vi "File Load Dialog.vi"(6 "cycle range":u16=720, 8 "error in (no error)":errorcluster, 11 "Node Ptr":T4 format="%.0x") -> (0 "error out":errorcluster, 1 "Position reference":T1, 2 "Cancelled":bool, 3 "Data":dbl[](array[numeric]))   [LabVIEW 2013, in "Engine Simulation Toolkit System Explorer.lvlib"]
uses:
  Engine Simulation Toolkit System Explorer.lvlib
  FPGA Mem Size.ctl
  Position Reference.ctl
  Data Replay Data Selection Method.ctl
  <vilib>/NI Veristand/Custom Device API/Custom Device Item Ref.ctl
  Data File Loader/File Interface.lvlib
  <vilib>/NI Veristand/Custom Device API/Custom Device API.lvlib
panel:
  in  "DispTwoRotations":bool
  in  "ReverseData":bool
  in  "Missing teeth location (degrees)":dbl=1.0 min=0.0
  in  "Samples":i32=1 min=1
  in  "File start offset":i32=1 min=0
  in  "Data Selection Method":T2
  in  "DataPlugin":u16(ring)
  out "Loaded samples":i32=1 min=1
  out "Loaded start offset":i32=1 min=0
  in  "Channel":u16(ring)
  in  "Selected File":path
  in  "Group":u16(ring)
  in  "FPGA memory size":T3=enum."16,384"
  in  "CycleAngle?":T1 caption="Position reference"
  in  "Cancel":bool
  in  "OK":bool
  out "Data Graph":waveform(dbl)(graph)
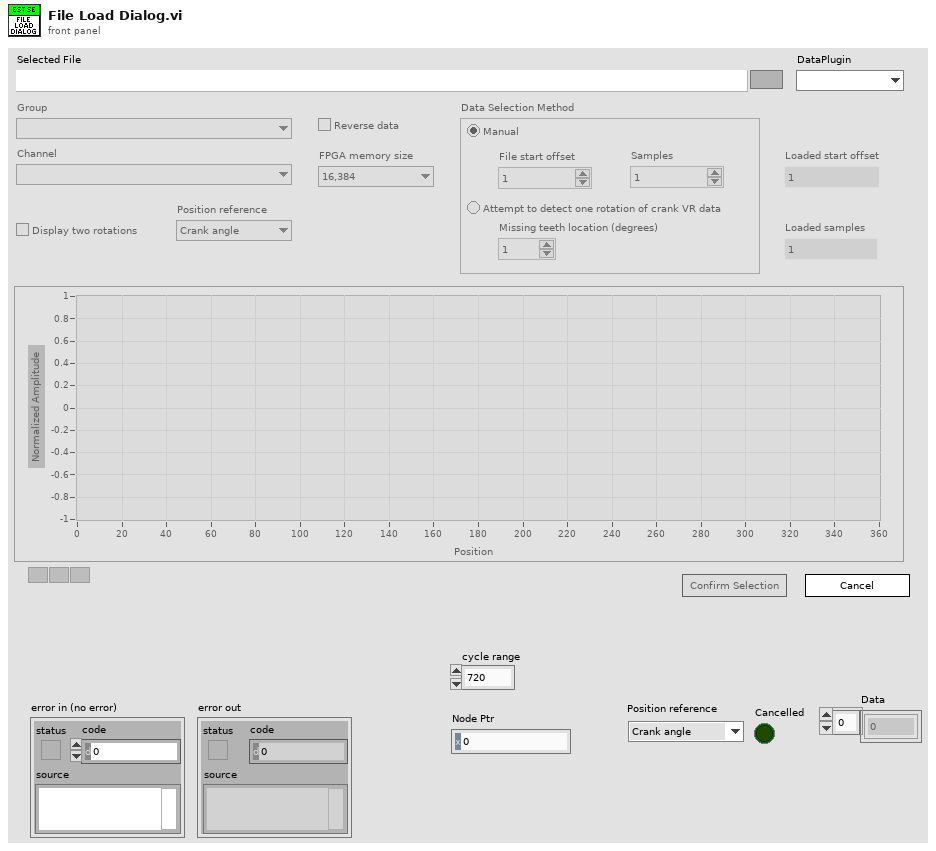
[diagram p1: front panel]
types:
  T1 = typedef "Engine Simulation Toolkit System Explorer.lvlib/Position Reference.ctl" = enum16{"Crank angle", "Cycle angle"}
  T2 = typedef "Engine Simulation Toolkit System Explorer.lvlib/Data Replay Data Selection Method.ctl" = enum32{"Manual", "AutoVRCrank"}
  T3 = typedef "Engine Simulation Toolkit System Explorer.lvlib/FPGA Mem Size.ctl" = enum16{"65,536", "32,768", "16,384", "8,192", "4,096", "2,048", "1,024"}
  T4 = typedef "Custom Device API.lvlib/Custom Device Item Ref.ctl" = u64
  T5 = typedef "Engine Simulation Toolkit System Explorer.lvlib/File Load Dialog.ctl" = cluster{"File":path, "Group":string, "Channel":string, "DataPlugin":string, "MissingTeeth":dbl, "ErrState":string, "File Selected":bool, "Data Selection Method":T2, "Offset":i32, "Length":i32, "DataPlugins Info":T6[], "Controls":refnum<vi>[], "File Ref":refnum<k20>, "Groups":string[], "Channels":string[], "Groups Refs":refnum<k20>[], "Channel Refs":refnum<k20>[], "Cancelled":bool, "Position reference":T1, "FPGA memory size":T3, "GroupRef":refnum<k20>, "ChanRef":refnum<k20>, "Data":dbl[], "ReverseData":bool, "DispTwoRotations":bool, "cycle range":u16}
  T6 = typedef "usiPluginInformation.ctl" = cluster{"name":string, "version":string, "type":string, "read-only?":bool, "extensions":string[]}
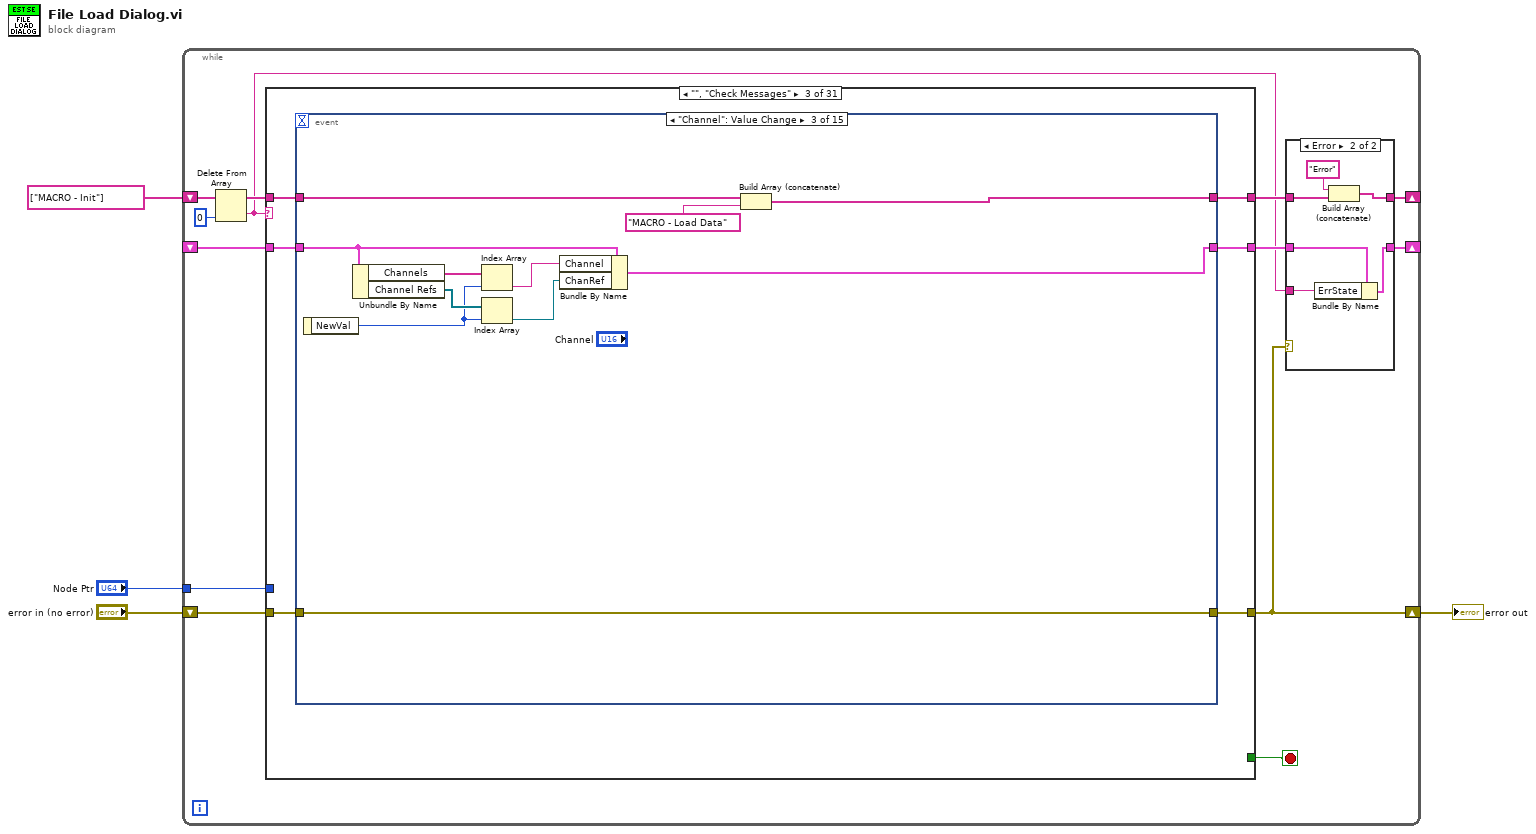
[diagram p0: block diagram]
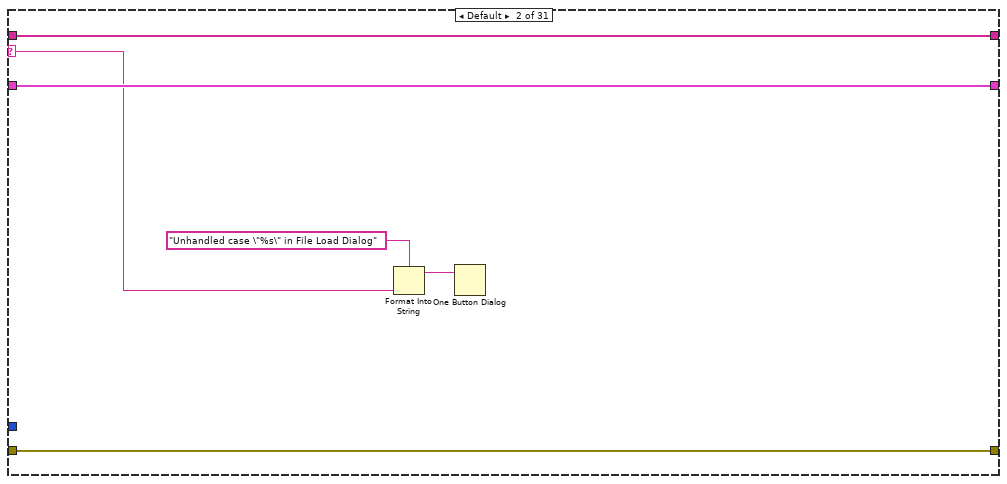
[diagram p4: hidden frame]
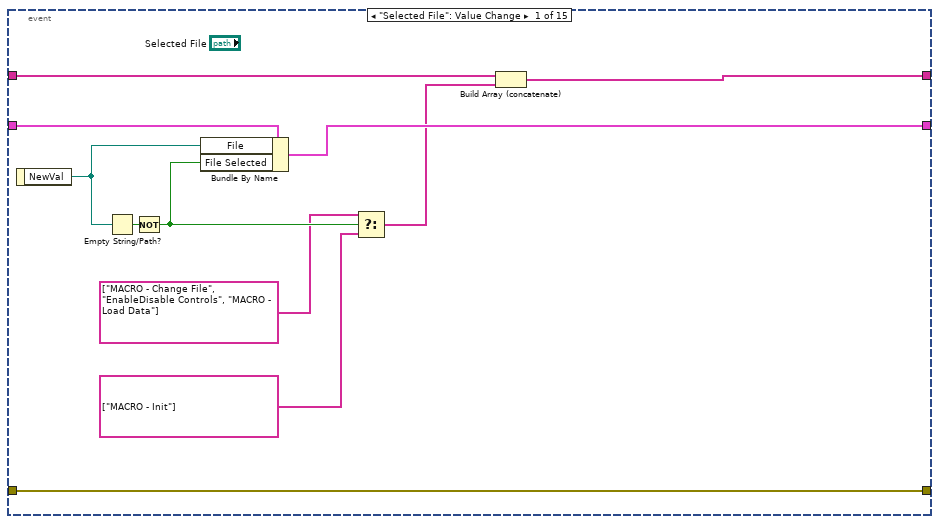
[diagram p5: hidden frame]
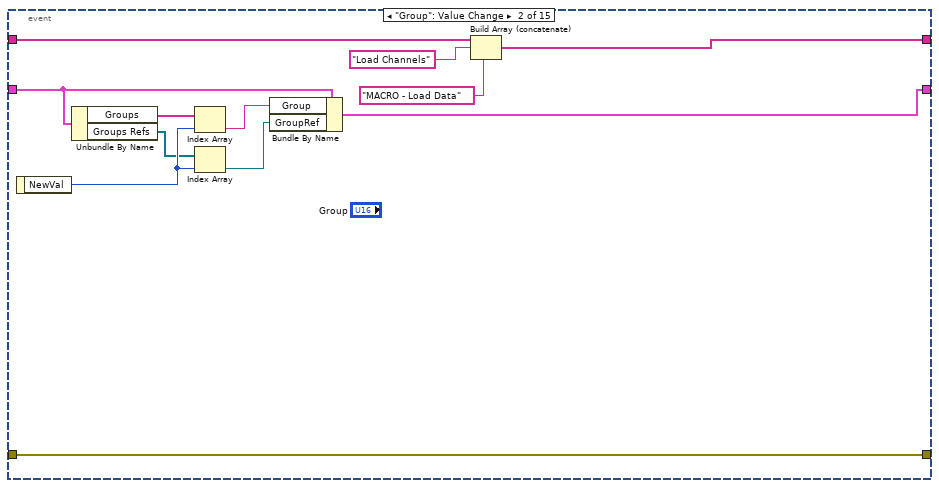
[diagram p6: hidden frame]
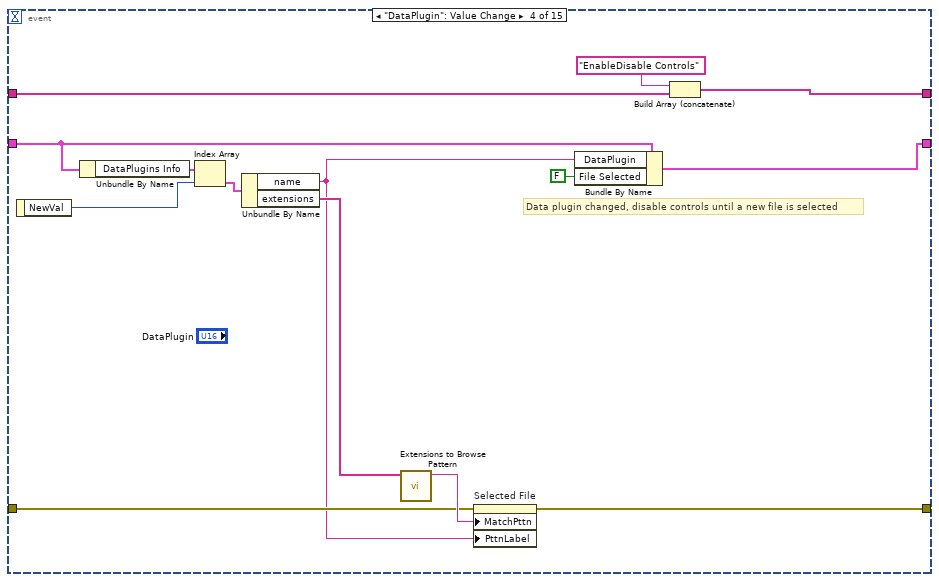
[diagram p7: hidden frame]
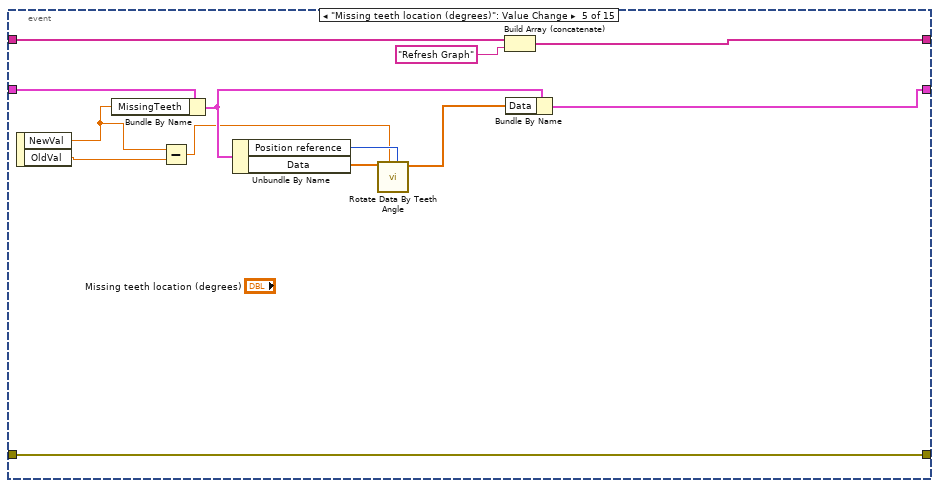
[diagram p8: hidden frame]
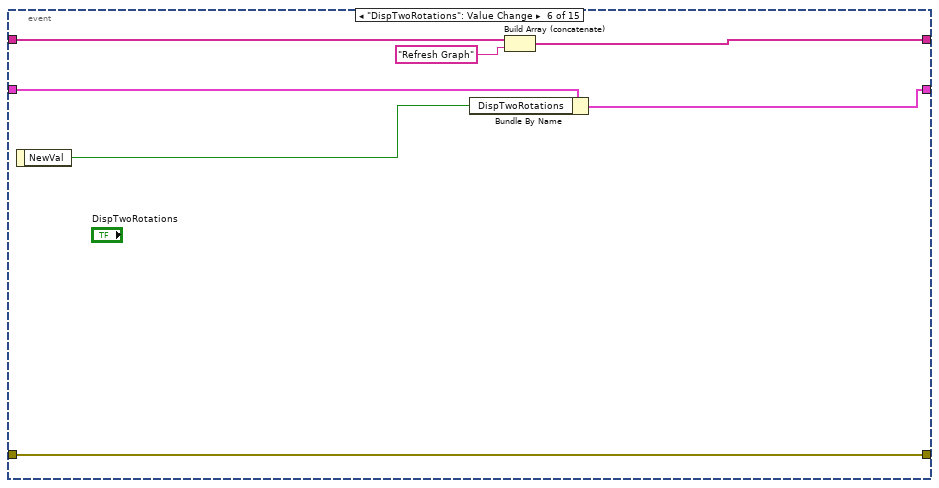
[diagram p9: hidden frame]
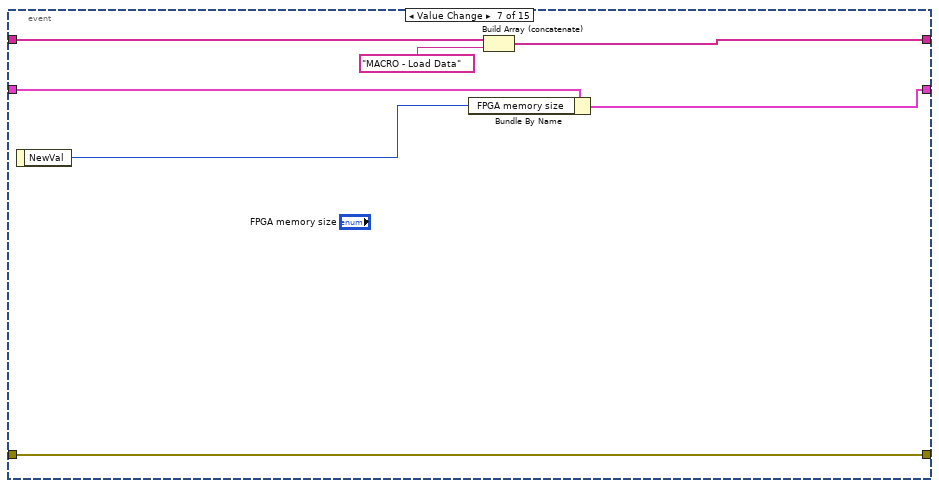
[diagram p10: hidden frame]
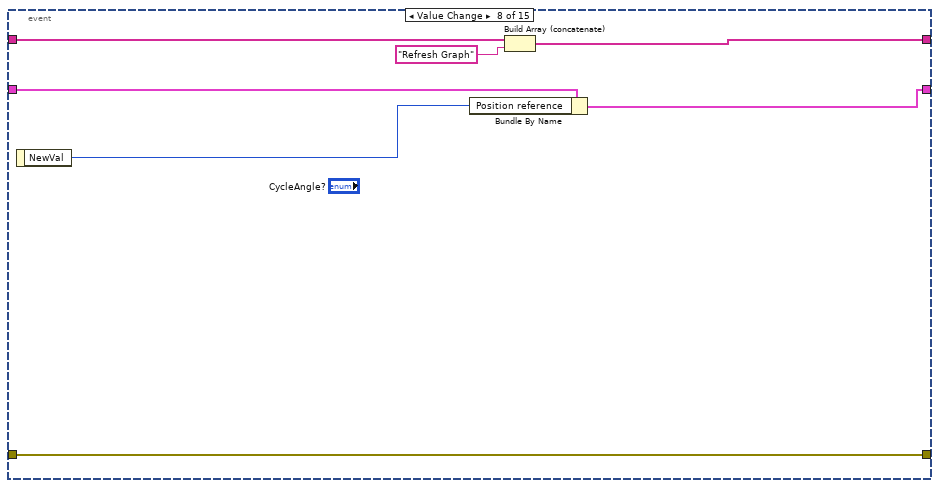
[diagram p11: hidden frame]
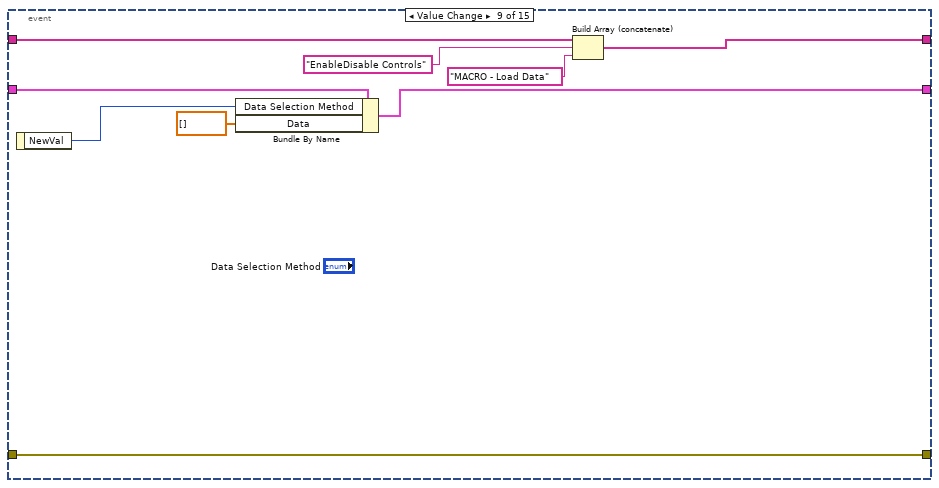
[diagram p12: hidden frame]
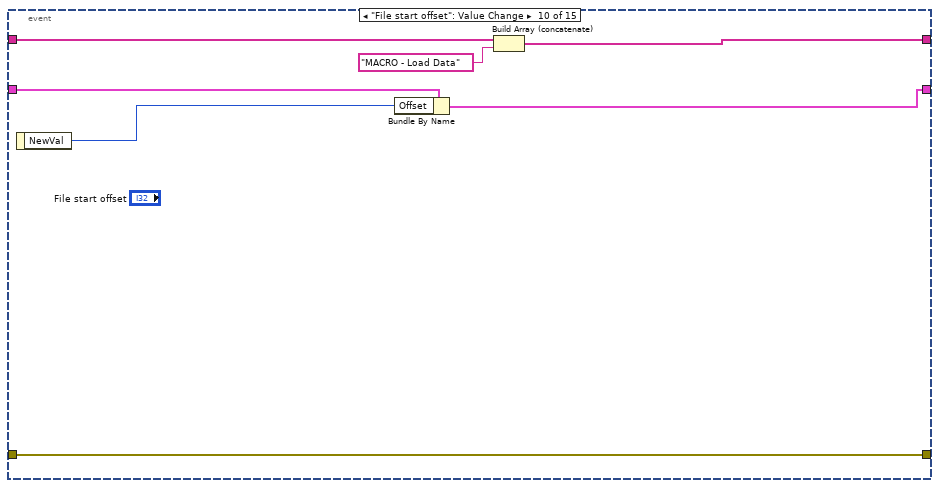
[diagram p13: hidden frame]
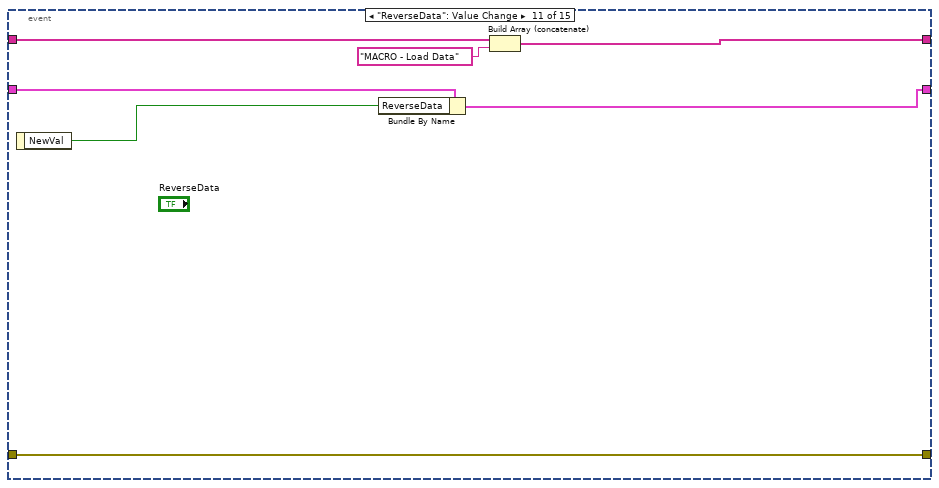
[diagram p14: hidden frame]
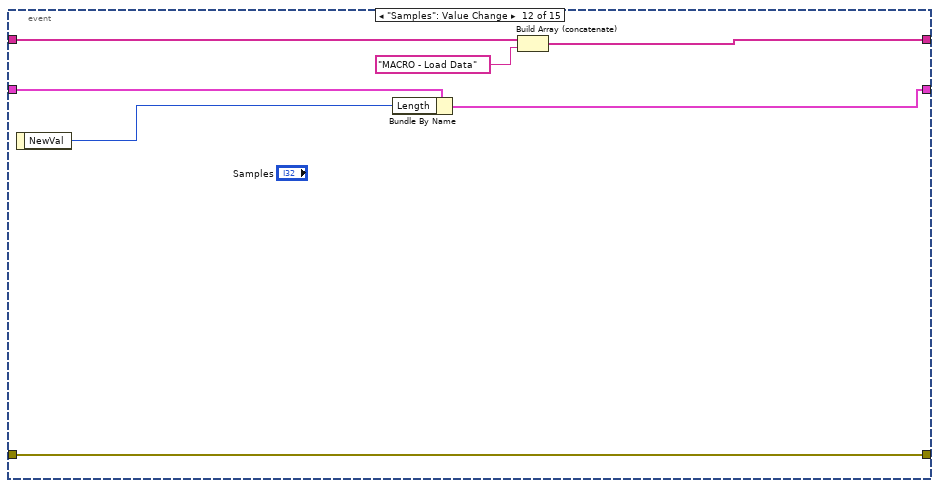
[diagram p15: hidden frame]
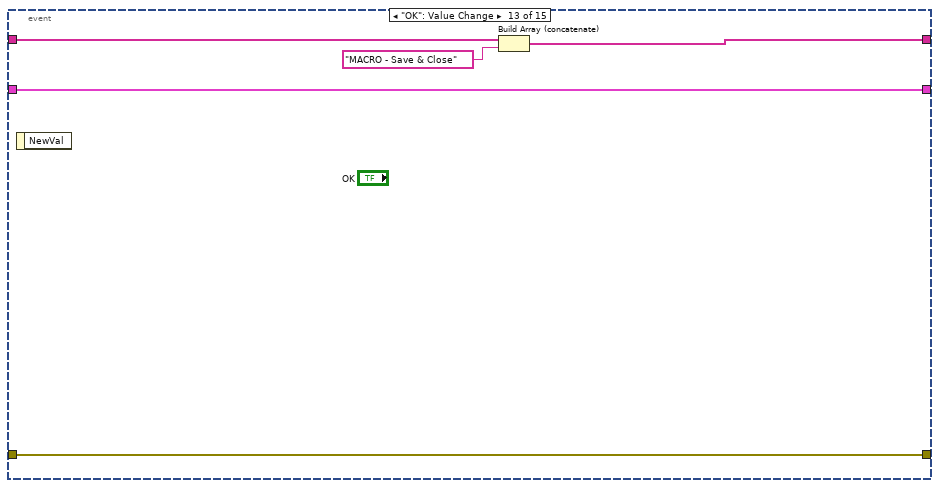
[diagram p16: hidden frame]
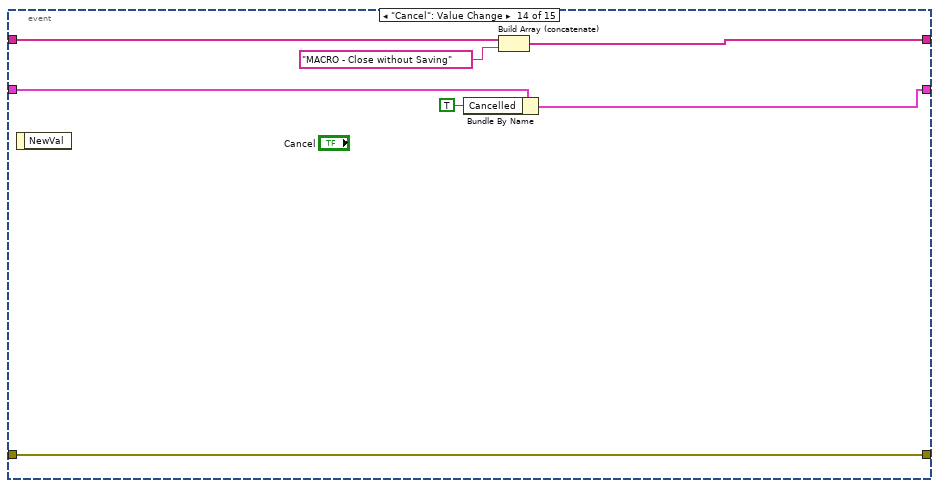
[diagram p17: hidden frame]
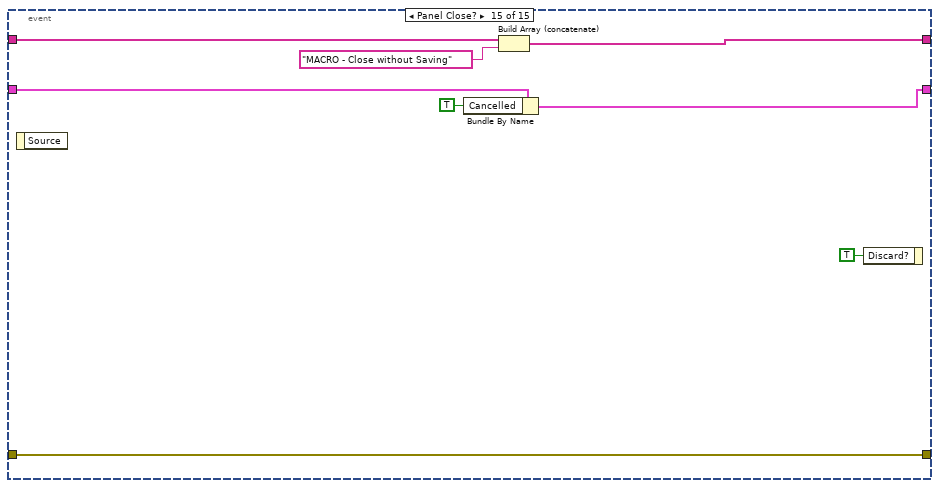
[diagram p18: hidden frame]
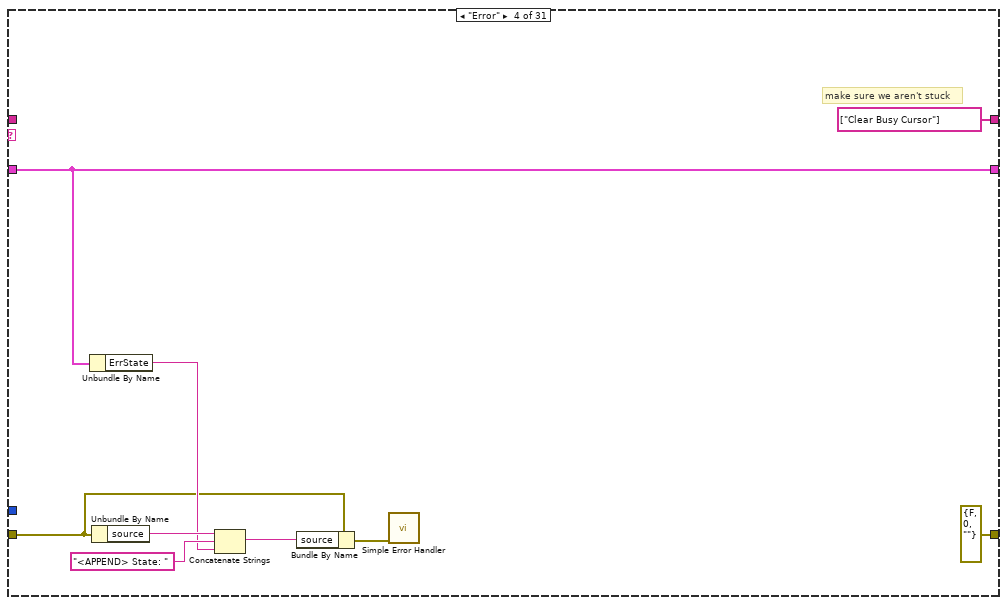
[diagram p19: hidden frame]
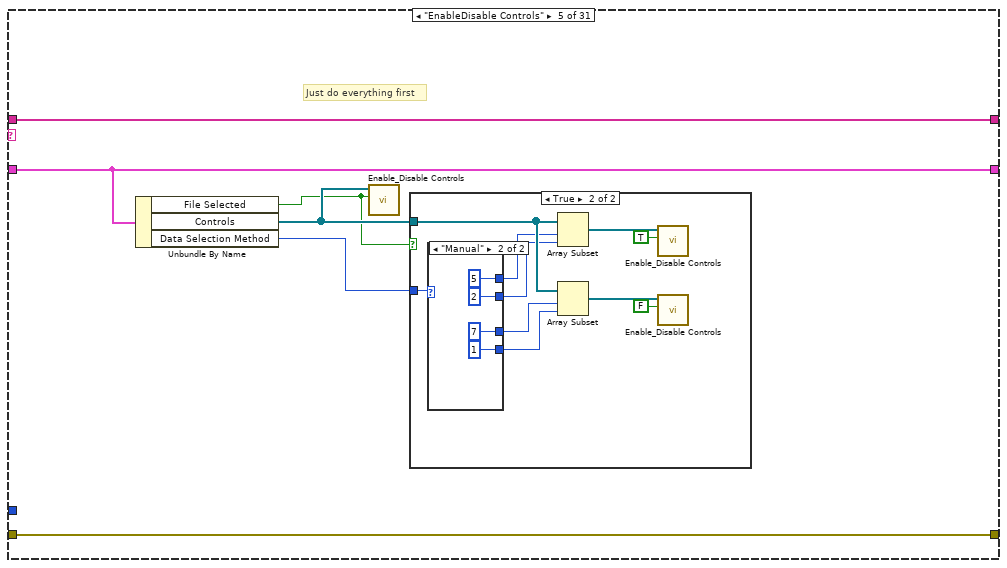
[diagram p20: hidden frame]
diagram:
  n1 = while {
    tunnel: "Node Ptr" -> [w16]
    shift-right: [w12] -> _
    shift-left: string[] ["MACRO - Init"] -> [w15]
    shift-right: [w10] -> _
    shift-left: _ -> [w9]
    shift-right: [w8] -> w1
    shift-left: "error in (no error)" -> [w17]
    stop <- w7 stop-if-true
    n2 = Delete From Array(array=w15, index=0) -> (deleted portion=w5:string, array with subset deleted=w14:string[])  [unwired: 1 in]
    n3 = case shown="\"\", \"Check Messages\"" w5 {
      selector: w5 -> [_ w29 _ _ _ _ _ _ _ _ _ _ _ _ _ _ _ _ _ _ _ _ _ _ _ _ _ _ _ _ _]
      tunnel: w17 -> [w26 w32 w35 w175 w186 w207 w212 w221 w223 w233 w239 w260 w275 w293 w313 w339 w345 w351 w358 w360 w366 w371 w376 w381 w386 w388 w398 w421 w449 w483 w493]
      tunnel: w16 -> [_ _ _ _ _ _ _ _ _ _ _ _ _ _ _ _ _ w349 _ _ _ _ _ _ _ _ w397 _ _ _ _]
      tunnel: w14 -> [w28 w34 w39 _ w187 w209 w214 w222 w225 w234 w243 w252 w276 w294 w314 w340 w347 w352 w359 w362 w364 w369 w374 w379 w384 w390 w395 w431 w444 w486 w494]
      tunnel: [w28 w34 w40 string[] ["Clear Busy Cursor"] w187 w209 w214 w222 w225 w234 w243 w249 w276 w294 w303 w340 w347 w352 w359 w362 w363 w368 w373 w378 w383 w390 w395 w401 w445 w486 w494] -> w13
      tunnel: [w27 w33 w38 w180 w185 w208 w213 w220 w224 w226 w241 w254 w267 w285 w308 w327 w346 w348 w356 w361 w367 w372 w377 w382 w387 w389 w393 w415 w443 w484 w490] -> w11
      tunnel: [w26 w32 w36 errorcluster {"status"=FALSE, "code"=0, "source"=""} ("error out") w186 w206 w211 w221 w223 w232 w240 w253 w275 w293 w307 w333 w345 w350 w358 w360 w366 w371 w376 w381 w386 w388 w396 w417 w448 w483 w488] -> w8
      tunnel: w9 -> [w27 w33 w37 w180 w185 w208 w213 w220 w224 w228 w242 w255 w272 w290 w309 w329 w346 w348 w356 w361 w367 w372 w377 w382 w387 w389 _ w415 w442 w485 w492]
      tunnel: [_ _ _ _ _ _ _ _ _ _ _ _ _ _ _ _ _ _ TRUE _ _ _ _ _ _ _ _ _ _ _ _] -> w7
      frame "<------------------ System ------------------>" {
      }
      frame Default {
        n4 = Format Into String(format string="Unhandled case \"%s\" in File Load Dialog", w29) -> (resulting string=w30:string)  [unwired: 2 in, 1 out]
        n5 = One Button Dialog(message=w30) -> ()  [unwired: 1 in, 1 out]
      }
      frame "", "Check Messages" {
        n6 = event shown="[2] \"Channel\": Value Change" {
          selector: _ -> [_ _ _ _ _ _ _ _ _ _ _ _ _ _ _]
          dyn-events: _ -> [_ _ _ _ _ _ _ _ _ _ _ _ _ _ _]
          timeout: _ -> [_ _ _ _ _ _ _ _ _ _ _ _ _ _ _]
          tunnel: [w47 w57 w65 w76 w93 w105 w110 w119 w126 w133 w140 w147 w154 w161 w169] -> w40
          tunnel: w39 -> [w51 w63 w69 w85 w101 w108 w111 w122 w131 w138 w145 w152 w157 w164 w172]
          tunnel: [w49 w61 w73 w88 w95 w106 w114 w120 w128 w135 w142 w149 w156 w159 w167] -> w38
          tunnel: w37 -> [w50 w60 w72 w87 w99 w103 w113 w117 w129 w137 w144 w151 w156 w163 w171]
          tunnel: [w48 w62 w74 w80 w100 w107 w115 w121 w130 w136 w143 w150 w155 w162 w170] -> w36
          tunnel: w35 -> [w48 w62 w74 w81 w100 w107 w115 w121 w130 w136 w143 w150 w155 w162 w170]
          event "Selected File": Value Change {
            n7 = event-data() -> ("NewVal"=w46:path)  [unwired: 1 in]
            n8 = Empty String/Path?(string/path=w46) -> (empty?=w45:bool)
            n9 = Not(x=w45) -> (.not. x?=w44:bool)
            n10 = Bundle By Name(cluster=w50, "File"=w46, "File Selected"=w44) -> (w49:T5)
            n11 = Select(t=string[] ["MACRO - Change File", "EnableDisable Controls", "MACRO - Load Data"], s=w44, f=string[] ["MACRO - Init"]) -> (s? t:f=w42:string[])
            n12 = Build Array (concatenate)(w51, w42) -> (w47:string[])
          }
          event "Group": Value Change {
            n13 = event-data() -> ("NewVal"=w55:u16)  [unwired: 1 in]
            n14 = Unbundle By Name(w60) -> ("Groups"=w59:string[], "Groups Refs"=w54:refnum<k20>[])
            n15 = Index Array(array=w59, index=w55) -> (element=w58:string)
            n16 = Index Array(array=w54, index=w55) -> (element=w53:refnum<k20>)
            n17 = Bundle By Name(cluster=w60, "Group"=w58, "GroupRef"=w53) -> (w61:T5)
            n18 = Build Array (concatenate)(w63, "Load Channels", "MACRO - Load Data") -> (w57:string[])
          }
          event "Channel": Value Change {
            n19 = event-data() -> ("NewVal"=w67:u16)  [unwired: 1 in]
            n20 = Unbundle By Name(w72) -> ("Channels"=w71:string[], "Channel Refs"=w68:refnum<k20>[])
            n21 = Index Array(array=w71, index=w67) -> (element=w70:string)
            n22 = Index Array(array=w68, index=w67) -> (element=w66:refnum<k20>)
            n23 = Bundle By Name(cluster=w72, "Channel"=w70, "ChanRef"=w66) -> (w73:T5)
            n24 = Build Array (concatenate)(w69, "MACRO - Load Data") -> (w65:string[])
          }
          event "DataPlugin": Value Change {
            # "Data plugin changed, disable controls until a new file is selected"
            n25 = event-data() -> ("NewVal"=w83:u16)  [unwired: 1 in]
            n26 = Unbundle By Name(w87) -> ("DataPlugins Info"=w86:T6[])
            n27 = Index Array(array=w86, index=w83) -> (element=w84:T6)
            n28 = Unbundle By Name(w84) -> ("name"=w78:string, "extensions"=w79:string[])
            n29 = call "Extensions to Browse Pattern.vi"("extensions"=w79) -> ("spreadsheet string"=w82:string)  [unwired: 10 in]
            n30 = property on="Selected File" class="Path"(error in=w81, "MatchPttn"=w82, "PttnLabel"=w78) -> (error out=w80:errorcluster)  [unwired: 1 in, 1 out]
            n31 = Bundle By Name(cluster=w87, "DataPlugin"=w78, "File Selected"=FALSE) -> (w88:T5)
            n32 = Build Array (concatenate)("EnableDisable Controls", w85) -> (w76:string[])
          }
          event "Missing teeth location (degrees)": Value Change {
            n33 = event-data() -> ("NewVal"=w91:dbl, "OldVal"=w90:dbl)  [unwired: 1 in]
            n34 = Bundle By Name(cluster=w99, "MissingTeeth"=w91) -> (w98:T5)
            n35 = Subtract(x=w91, y=w90) -> (x-y=w89:dbl)
            n36 = Unbundle By Name(w98) -> ("Position reference"=w96:T1, "Data"=w97:dbl[])
            n37 = call "Rotate Data By Teeth Angle.vi"("Position reference"=w96, "Missing Tooth Angle"=w89, "One VR Crank Period"=w97) -> ("Rotated to desired angle"=w94:dbl[])  [unwired: 8 in]
            n38 = Build Array (concatenate)(w101, "Refresh Graph") -> (w93:string[])
            n39 = Bundle By Name(cluster=w98, "Data"=w94) -> (w95:T5)
          }
          event "DispTwoRotations": Value Change {
            n40 = event-data() -> ("NewVal"=w102:bool)  [unwired: 1 in]
            n41 = Bundle By Name(cluster=w103, "DispTwoRotations"=w102) -> (w106:T5)
            n42 = Build Array (concatenate)(w108, "Refresh Graph") -> (w105:string[])
          }
          event Value Change {
            n43 = event-data() -> ("NewVal"=w112:T3)  [unwired: 1 in]
            n44 = Bundle By Name(cluster=w113, "FPGA memory size"=w112) -> (w114:T5)
            n45 = Build Array (concatenate)(w111, "MACRO - Load Data") -> (w110:string[])
          }
          event Value Change {
            n46 = event-data() -> ("NewVal"=w116:T1)  [unwired: 1 in]
            n47 = Bundle By Name(cluster=w117, "Position reference"=w116) -> (w120:T5)
            n48 = Build Array (concatenate)(w122, "Refresh Graph") -> (w119:string[])
          }
          event Value Change {
            n49 = event-data() -> ("NewVal"=w127:T2)  [unwired: 1 in]
            n50 = Bundle By Name(cluster=w129, "Data Selection Method"=w127, "Data"=dbl[] []) -> (w128:T5)
            n51 = Build Array (concatenate)(w131, "EnableDisable Controls", "MACRO - Load Data") -> (w126:string[])
          }
          event "File start offset": Value Change {
            n52 = event-data() -> ("NewVal"=w134:i32)  [unwired: 1 in]
            n53 = Bundle By Name(cluster=w137, "Offset"=w134) -> (w135:T5)
            n54 = Build Array (concatenate)(w138, "MACRO - Load Data") -> (w133:string[])
          }
          event "ReverseData": Value Change {
            n55 = event-data() -> ("NewVal"=w141:bool)  [unwired: 1 in]
            n56 = Bundle By Name(cluster=w144, "ReverseData"=w141) -> (w142:T5)
            n57 = Build Array (concatenate)(w145, "MACRO - Load Data") -> (w140:string[])
          }
          event "Samples": Value Change {
            n58 = event-data() -> ("NewVal"=w148:i32)  [unwired: 1 in]
            n59 = Bundle By Name(cluster=w151, "Length"=w148) -> (w149:T5)
            n60 = Build Array (concatenate)(w152, "MACRO - Load Data") -> (w147:string[])
          }
          event "OK": Value Change {
            n61 = event-data() -> ()  [unwired: 1 in, 1 out]
            n62 = Build Array (concatenate)(w157, "MACRO - Save & Close") -> (w154:string[])
          }
          event "Cancel": Value Change {
            n63 = event-data() -> ()  [unwired: 1 in, 1 out]
            n64 = Bundle By Name(cluster=w163, "Cancelled"=TRUE) -> (w159:T5)
            n65 = Build Array (concatenate)(w164, "MACRO - Close without Saving") -> (w161:string[])
          }
          event Panel Close? {
            n66 = event-data() -> ()  [unwired: 1 in, 1 out]
            n67 = Bundle By Name(cluster=w171, "Cancelled"=TRUE) -> (w167:T5)
            n68 = Build Array (concatenate)(w172, "MACRO - Close without Saving") -> (w169:string[])
            n69 = event-data("Discard?"=TRUE) -> ()  [unwired: 1 in, 1 out]
          }
        }
      }
      frame "Error" {
        # "make sure we aren't stuck"
        n70 = Unbundle By Name(w180) -> ("ErrState"=w177:string)
        n71 = Unbundle By Name(w175) -> ("source"=w179:string)
        n72 = Concatenate Strings(w179, "<APPEND> State: " ("string"), w177) -> (w176:string)
        n73 = Bundle By Name(cluster=w175, "source"=w176) -> (w174:errorcluster)
        n74 = call <vilib>:"Simple Error Handler.vi"("error in (no error)"=w174) -> ()  [unwired: 4 in, 5 out]
      }
      frame "EnableDisable Controls" {
        # "Just do everything first"
        n75 = Unbundle By Name(w185) -> ("File Selected"=w182:bool, "Controls"=w183:refnum<vi>[], "Data Selection Method"=w184:T2)
        n76 = call "Enable_Disable Controls.vi"("Enable?"=w182, "Controls"=w183) -> ()  [unwired: 10 in]
        n77 = case shown="True" w182 {
          tunnel: w184 -> [_ w197]
          tunnel: w183 -> [_ w196]
          frame False {
          }
          frame True {
            n78 = case shown="\"Manual\"" w197 {
              tunnel: [1 ("length") 2 ("length")] -> w195
              tunnel: [7 ("index") 5 ("index")] -> w194
              tunnel: [5 ("index") 7 ("index")] -> w189
              tunnel: [2 ("length") 1 ("length")] -> w188
              frame "AutoVRCrank" {
              }
              frame "Manual" {
              }
            }
            n79 = Array Subset(array=w196, index=w194, length=w195) -> (w193:refnum<vi>[])
            n80 = Array Subset(array=w196, index=w189, length=w188) -> (w190:refnum<vi>[])
            n81 = call "Enable_Disable Controls.vi"("Enable?"=TRUE, "Controls"=w193) -> ()  [unwired: 10 in]
            n82 = call "Enable_Disable Controls.vi"("Enable?"=FALSE, "Controls"=w190) -> ()  [unwired: 10 in]
          }
        }
      }
      frame "Set Busy Cursor" {
        n83 = call <vilib>:"Set Busy.vi"("error in (no error)"=w207) -> ("error out"=w206:errorcluster)  [unwired: 9 in, 1 out]
      }
      frame "Clear Busy Cursor" {
        n84 = call <vilib>:"Unset Busy.vi"() -> ("error out"=w210:errorcluster)  [unwired: 11 in]
        n85 = Merge Errors(w210, w212) -> (w211:errorcluster)
      }
      frame "Refresh Graph" {
        n86 = Unbundle By Name(w220) -> ("Data"=w219:dbl[], "Position reference"=w218:T1, "DispTwoRotations"=w216:bool, "cycle range"=w215:u16)
        n87 = call "Data Replay DBLs to Waveform.vi"("cycle range"=w215, "display two rotations? (F)"=w216, "Position reference"=w218, "Data"=w219) -> ("waveform"=→"Data Graph":waveform(dbl))  [unwired: 7 in]
      }
      frame "<------------- File Interaction------------->" {
      }
      frame "Open File" {
        n88 = Unbundle By Name(w228) -> ("File"=w231:path, "DataPlugin"=w230:string)
        n89 = case shown="\"CSV\"" w230 {
          tunnel: [_ "<allnumericfloat64>yes</allnumericfloat64>"] -> w229
          frame Default {
          }
          frame "CSV" {
            # "Disables auto detect of data type. Forces dbl"
          }
        }
        n90 = call "Open Data File.vi"("error in (no error)"=w233, "Additional parameters"=w229, "Data Plugin"=w230, "File Path"=w231) -> ("error out"=w232:errorcluster, "File Ref"=w227:refnum<k20>)  [unwired: 6 in]
        n91 = Bundle By Name(cluster=w228, "File Ref"=w227) -> (w226:T5)
      }
      frame "Close File" {
        n92 = Unbundle By Name(w242) -> ("File Ref"=w237:refnum<k20>)
        n93 = Not A Number/Path/Refnum?(number/path/refnum=w237) -> (NaN/Path/Refnum?=w236:bool)
        n94 = case shown="False" w236 {
          tunnel: [w246 w247] -> w240
          tunnel: w239 -> [w245 w247]
          tunnel: w237 -> [w244 _]
          frame False {
            n95 = call "Close Data File.vi"("error in (no error)"=w245, "File Ref"=w244) -> ("error out"=w246:errorcluster)  [unwired: 9 in]
          }
          frame True {
          }
        }
        n96 = Bundle By Name(cluster=w242, "File Ref"=refnum<k0> refnum) -> (w241:T5)
      }
      frame "Load Groups" {
        n97 = Unbundle By Name(w255) -> ("File Ref"=w259:refnum<k20>)
        n98 = call "Get Channel Groups.vi"("error in (no error)"=w260, "File Ref in"=w259) -> ("error out"=w258:errorcluster, "Channel Groups"=w257:refnum<k20>[])  [unwired: 7 in, 1 out]
        n99 = for {
          shift-right: [w263] -> w256
          shift-left: w258 -> [w265]
          tunnel: w257 -> [w264] mode=indexing
          tunnel: [w262] -> w251 mode=indexing
          tunnel: [w261] -> w250 mode=indexing
          n100 = call "Get Object Name.vi"("error in (no error)"=w265, "Storage Object in"=w264) -> ("error out"=w263:errorcluster, "Name"=w262:string, "Storage Object out"=w261:refnum<k20>)  [unwired: 7 in]
        }
        n101 = Build Array (concatenate)("Validate Group", w252) -> (w249:string[])
        n102 = property on="Group" class="Ring (strict)"(error in=w256, "Strings []"=w251) -> (error out=w253:errorcluster)  [unwired: 1 in, 1 out]
        n103 = Bundle By Name(cluster=w255, "Groups"=w251, "Groups Refs"=w250) -> (w254:T5)
      }
      frame "Validate Group" {
        n104 = Unbundle By Name(w272) -> ("Groups"=w271:string[], "Group"=w274:string, "Groups Refs"=w269:refnum<k20>[])
        n105 = Search 1D Array(1D array=w271, element=w274) -> (index of element=w273:i32)  [unwired: 1 in]
        n106 = case shown="-1" w273 {
          selector: w273 -> [_ w283]
          tunnel: w272 -> [w281 w282]
          tunnel: w271 -> [w280 _]
          tunnel: [w278 w282] -> w270
          tunnel: [w277 w283] -> w266
          frame -1 {
            w277 = 0
            # "not found. use first"
            n107 = Index Array(array=w280, index=w277) -> (element=w279:string)
            n108 = Bundle By Name(cluster=w281, "Group"=w279) -> (w278:T5)
          }
          frame Default {
            # "Found, set ref"
          }
        }
        n109 = Index Array(array=w269, index=w266) -> (element=w268:refnum<k20>)
        n110 = local write "Group"(w266) -> ()
        n111 = Bundle By Name(cluster=w270, "GroupRef"=w268) -> (w267:T5)
      }
      frame "Validate Channel" {
        n112 = Unbundle By Name(w290) -> ("Channels"=w289:string[], "Channel"=w292:string, "Channel Refs"=w287:refnum<k20>[])
        n113 = Search 1D Array(1D array=w289, element=w292) -> (index of element=w291:i32)  [unwired: 1 in]
        n114 = case shown="-1" w291 {
          selector: w291 -> [_ w301]
          tunnel: w290 -> [w299 w300]
          tunnel: w289 -> [w298 _]
          tunnel: [w296 w300] -> w288
          tunnel: [w295 w301] -> w284
          frame -1 {
            w295 = 0
            # "not found. use first"
            n115 = Index Array(array=w298, index=w295) -> (element=w297:string)
            n116 = Bundle By Name(cluster=w299, "Channel"=w297) -> (w296:T5)
          }
          frame Default {
            # "Found, set ref"
          }
        }
        n117 = Index Array(array=w287, index=w284) -> (element=w286:refnum<k20>)
        n118 = local write "Channel"(w284) -> ()
        n119 = Bundle By Name(cluster=w288, "ChanRef"=w286) -> (w285:T5)
      }
      frame "Load Channels" {
        n120 = Unbundle By Name(w309) -> ("GroupRef"=w306:refnum<k20>)
        n121 = call "Get Channels.vi"("error in (no error)"=w313, "Channel Group in"=w306) -> ("error out"=w312:errorcluster, "Channels"=w311:refnum<k20>[])  [unwired: 7 in, 1 out]
        n122 = for {
          shift-right: [w317] -> w310
          shift-left: w312 -> [w319]
          tunnel: w311 -> [w318] mode=indexing
          tunnel: [w316] -> w305 mode=indexing
          tunnel: [w315] -> w304 mode=indexing
          n123 = call "Get Object Name.vi"("error in (no error)"=w319, "Storage Object in"=w318) -> ("error out"=w317:errorcluster, "Name"=w316:string, "Storage Object out"=w315:refnum<k20>)  [unwired: 7 in]
        }
        n124 = Build Array (concatenate)("Validate Channel", w314) -> (w303:string[])
        n125 = Bundle By Name(cluster=w309, "Channels"=w305, "Channel Refs"=w304) -> (w308:T5)
        n126 = property on="Channel" class="Ring (strict)"(error in=w310, "Strings []"=w305) -> (error out=w307:errorcluster)  [unwired: 1 in, 1 out]
      }
      frame "Load Data" {
        n127 = Unbundle By Name(w329) -> ("Position reference"=w330:T1, "MissingTeeth"=w331:dbl, "ReverseData"=w320:bool, "ChanRef"=w336:refnum<k20>, "Offset"=w334:i32, "Length"=w335:i32, "Data Selection Method"=w322:T2, "FPGA memory size"=w338:T3)
        n128 = call "Memory Size Enum to Numeric.vi"("error in (no error)"=w339, "FPGA Memory Size"=w338) -> ("error out"=w337:errorcluster, "Numeric"=w325:i32)  [unwired: 8 in]
        n129 = case shown="\"AutoVRCrank\"" w322 {
          tunnel: [w342 0 ("Count (0: Read All)")] -> w332
          tunnel: [w341 0 ("index")] -> w321
          tunnel: w335 -> [w342 _]
          tunnel: w334 -> [w341 _]
          frame "Manual", Default {
          }
          frame "AutoVRCrank" {
          }
        }
        n130 = call "Get Channel Data.vi"("error in"=w337, "Count (0: Read All)"=w332, "index"=w321, "Channel in"=w336) -> ("error out"=w333:errorcluster, "Signal"=w326:dbl[])  [unwired: 5 in, 1 out]
        n131 = call "Select Data Subset From Loaded Data.vi"("Position reference"=w330, "Memory Size as number"=w325, "MissingTeeth"=w331, "ReverseData"=w320, "Offset"=w321, "Data Selection Method"=w322, "Signal"=w326) -> ("Selected Length"=→"Loaded samples":i32, "Selected Offset"=→"Loaded start offset":i32, "Resampled Data"=w328:dbl[])  [unwired: 2 in]
        n132 = Bundle By Name(cluster=w329, "Data"=w328) -> (w327:T5)
      }
      frame "<------------------ Shut Down ------------------>" {
      }
      frame "Save Data" {
        n133 = call "Save File Load Dialog Data.vi"("error in (no error)"=w351, "FileDialog"=w348, "Node Ptr"=w349) -> ("error out"=w350:errorcluster)  [unwired: 8 in]
      }
      frame "Exit" {
        n134 = Unbundle By Name(w356) -> ("Cancelled"=→"Cancelled":bool, "Data"=→"Data":dbl[], "Position reference"=→"Position reference":T1)
      }
      frame "<------------------ Macros ------------------>" {
      }
      frame "MACRO - Init" {
        n135 = Build Array (concatenate)(string[] ["Set Busy Cursor", "Init Data", "Get DataPlugin List", "Validate File Existis", "Get Refs", "Init UI", "EnableDisable Controls", "Clear Busy Cursor"], w364) -> (w363:string[])
      }
      frame "MACRO - Save & Close" {
        n136 = Build Array (concatenate)(string[] ["Close File", "Save Data", "Exit"], w369) -> (w368:string[])
      }
      frame "MACRO - Close without Saving" {
        n137 = Build Array (concatenate)(string[] ["Close File", "Exit"], w374) -> (w373:string[])
      }
      frame "MACRO - Change File" {
        n138 = Build Array (concatenate)(string[] ["Set Busy Cursor", "Close File", "Open File", "Load Groups", "Load Channels", "Clear Busy Cursor"], w379) -> (w378:string[])
      }
      frame "MACRO - Load Data" {
        n139 = Build Array (concatenate)(string[] ["Set Busy Cursor", "Load Data", "Refresh Graph", "Clear Busy Cursor"], w384) -> (w383:string[])
      }
      frame "<------------------ Initialization ------------------>" {
      }
      frame "Init Data" {
        # "Clear graph"
        n140 = call "Init File Load Dialog Data.vi"("error in (no error)"=w398, "Node Ptr"=w397) -> ("error out"=w396:errorcluster, "FileDialog"=w394:T5)  [unwired: 8 in]
        n141 = local write "Data Graph"(waveform(dbl) {"t0"=timestamp(0 s since 1904-01-01), "dt"=1.0, "Y"=[]} ("Data Graph")) -> ()
        n142 = Bundle By Name(cluster=w394, "cycle range"="cycle range") -> (w393:T5)
      }
      frame "Init UI" {
        # "None of these are user controls"
        n143 = Unbundle By Name(w415) -> ("File Selected"=w400:bool, "Position reference"=w403:T1, "FPGA memory size"=w402:T3, "File"=w418:path, "MissingTeeth"=w430:dbl, "Data Selection Method"=w429:T2, "Offset"=w428:i32, "Length"=w427:i32, "ReverseData"=w404:bool, "DataPlugins Info"=w426:T6[], "DataPlugin"=w419:string)
        n144 = for {
          tunnel: w426 -> [w441] mode=indexing
          tunnel: [w440] -> w425 mode=indexing
          tunnel: [w438] -> w424 mode=indexing
          n145 = Unbundle By Name(w441) -> ("name"=w440:string, "extensions"=w439:string[])
          n146 = Bundle("extensions"=w439) -> (w438:cluster{"extensions":string[]})  [unwired: 1 in]
        }
        n147 = local write "CycleAngle?"(w403) -> ()
        n148 = local write "FPGA memory size"(w402) -> ()
        n149 = local write "Selected File"(w418) -> ()
        n150 = local write "Missing teeth location (degrees)"(w430) -> ()
        n151 = local write "Data Selection Method"(w429) -> ()
        n152 = local write "File start offset"(w428) -> ()
        n153 = local write "Samples"(w427) -> ()
        n154 = local write "ReverseData"(w404) -> ()
        n155 = Search 1D Array(1D array=w425, element=w419) -> (index of element=w416:i32)  [unwired: 1 in]
        n156 = case shown="False" w400 {
          tunnel: w431 -> [w432 w435]
          tunnel: [w432 w434] -> w401
          frame False {
          }
          frame True {
            n157 = Build Array (concatenate)("MACRO - Load Data", w435) -> (w434:string[])
          }
        }
        n158 = Index Array(array=w424, index=w416) -> (element=w423:cluster{"extensions":string[]})
        n159 = local write "DataPlugin"(w416) -> ()
        n160 = Unbundle(w423) -> ("extensions"=w422:string[])
        n161 = call "Extensions to Browse Pattern.vi"("extensions"=w422) -> ("spreadsheet string"=w420:string)  [unwired: 10 in]
        n162 = control-ref of="Cancelled"() -> (w413:refnum<vi>)
        n163 = control-ref of="error in (no error)"() -> (w407:refnum<vi>)
        n164 = control-ref of="error out"() -> (w406:refnum<vi>)
        n165 = control-ref of="cycle range"() -> (w399:refnum<vi>)
        n166 = control-ref of="Loaded samples"() -> (w410:refnum<vi>)
        n167 = control-ref of="Loaded start offset"() -> (w409:refnum<vi>)
        n168 = control-ref of="Node Ptr"() -> (w408:refnum<vi>)
        n169 = control-ref of="cycle angle"() -> (w412:refnum<vi>)
        n170 = control-ref of="Data"() -> (w411:refnum<vi>)
        n171 = property on="Selected File" class="Path"(error in=w421, "MatchPttn"=w420, "PttnLabel"=w419) -> (error out=w417:errorcluster)  [unwired: 1 in, 1 out]
        n172 = Build Array(w413, w412, w411, w399, w410, w409, w408, w407, w406) -> (w405:refnum<vi>[])
        n173 = for {
          tunnel: TRUE ("Skip When Tabbing") -> [w437]
          tunnel: w405 -> [w436] mode=indexing
          n174 = property on="Property Node" class="Ctl"(reference=w436, "SkipTabbing"=w437) -> ()  [unwired: 1 in, 2 out]
        }
      }
      frame "Validate File Existis" {
        n175 = Unbundle By Name(w442) -> ("File"=w447:path, "File Selected"=w446:bool)
        n176 = case shown="True" w446 {
          tunnel: w449 -> [w452 w463]
          tunnel: [w452 w462] -> w448
          tunnel: w447 -> [_ w453]
          tunnel: [w451 w458] -> w445
          tunnel: w444 -> [w451 w459]
          tunnel: [w450 w456] -> w443
          tunnel: w442 -> [w450 w457]
          frame False {
          }
          frame True {
            n177 = call <vilib>:"Check if File or Folder Exists.vi"("error in (no error)"=w463, "path"=w453) -> ("error out"=w462:errorcluster, "file or folder exists?"=w455:bool)  [unwired: 7 in, 1 out]
            n178 = Select(t=w453, s=w455, f=path "") -> (s? t:f=w460:path)
            n179 = case shown="False" w455 {
              tunnel: "MACRO - Change File" -> [_ w467]
              tunnel: w459 -> [w464 w466]
              tunnel: [w464 w465] -> w458
              frame False {
              }
              frame True {
                n180 = Build Array (concatenate)(w467, w466) -> (w465:string[])
              }
            }
            n181 = Bundle By Name(cluster=w457, "File Selected"=w455, "File"=w460) -> (w456:T5)
          }
        }
      }
      frame "Get Refs" {
        n182 = control-ref of="Group"() -> (w480:refnum<vi>)
        n183 = control-ref of="Channel"() -> (w479:refnum<vi>)
        n184 = control-ref of="Loaded start offset"() -> (w478:refnum<vi>)
        n185 = control-ref of="Loaded samples"() -> (w477:refnum<vi>)
        n186 = control-ref of="Data Selection Method"() -> (w476:refnum<vi>)
        n187 = control-ref of="File start offset"() -> (w475:refnum<vi>)
        n188 = control-ref of="Samples"() -> (w474:refnum<vi>)
        n189 = control-ref of="Missing teeth location (degrees)"() -> (w473:refnum<vi>)
        n190 = control-ref of="OK"() -> (w472:refnum<vi>)
        n191 = control-ref of="Data Graph"() -> (w471:refnum<vi>)
        n192 = control-ref of="ReverseData"() -> (w470:refnum<vi>)
        n193 = control-ref of="DispTwoRotations"() -> (w469:refnum<vi>)
        n194 = control-ref of="FPGA memory size"() -> (w482:refnum<vi>)
        n195 = control-ref of="CycleAngle?"() -> (w481:refnum<vi>)
        n196 = Build Array(w480, w479, w478, w477, w476, w475, w474, w473, w472, w471, w470, w469, w481, w482) -> (w468:refnum<vi>[])
        n197 = Bundle By Name(cluster=w485, "Controls"=w468) -> (w484:T5)
      }
      frame "Get DataPlugin List" {
        n198 = call <vilib>:"List DataPlugins.vi"("error in (no error)"=w493) -> ("DataPlugin information"=w489:T6[], "error out"=w491:errorcluster)  [unwired: 13 in]
        n199 = for {
          tunnel: w489 -> [w496] mode=indexing
          tunnel: [w495] -> w487 mode=indexing
          n200 = Unbundle By Name(w496) -> ("name"=w495:string)
        }
        n201 = Bundle By Name(cluster=w492, "DataPlugins Info"=w489) -> (w490:T5)
        n202 = property on="DataPlugin" class="Ring (strict)"(error in=w491, "Strings []"=w487) -> (error out=w488:errorcluster)  [unwired: 1 in, 1 out]
      }
    }
    n203 = case shown="Error" w8 {
      tunnel: w13 -> [w18 w25]
      tunnel: [w18 w23] -> w12
      tunnel: w11 -> [w19 w22]
      tunnel: [w19 w21] -> w10
      tunnel: w5 -> [_ w20]
      frame No Error {
      }
      frame Error {
        n204 = Bundle By Name(cluster=w22, "ErrState"=w20) -> (w21:T5)
        n205 = Build Array (concatenate)("Error", w25) -> (w23:string[])
      }
    }
  }
  "error out" <- w1
